vi "Read_ROI.vi"(8 "error in":errorcluster, 11 "Experiment folder path":path) -> (0 "error out":errorcluster, 2 "ROI setup":T1[](array[typedef]) {"ROI group ID" format="%#_6f"; "Laser Power (%)" format="%#_6f"; "Zoom" format="%#_6f"; "Frame Size" format="%#_6f"; "Number of lines" format="%#_6f"; "Composite ID" format="%#_6f"; "Angle (deg)" format="%#_6f"; "ROI Time (ns)" format="%#_6f"; "ROI ID" format="%#_6f"; "Pixels in ROI" format="%#_6f"; "ROI index" format="%#_6f"; "Z stop" format="%#_6f"; "Y stop" format="%#_6f"; "X stop" format="%#_6f"; "Z start" format="%#_6f"; "X start" format="%#_6f"; "Y start" format="%#_6f"})   [LabVIEW 2013]
uses:
  User Interface/Visualisation/Functional Imaging Viewer/Typedefs/ROI parameters data type.ctl
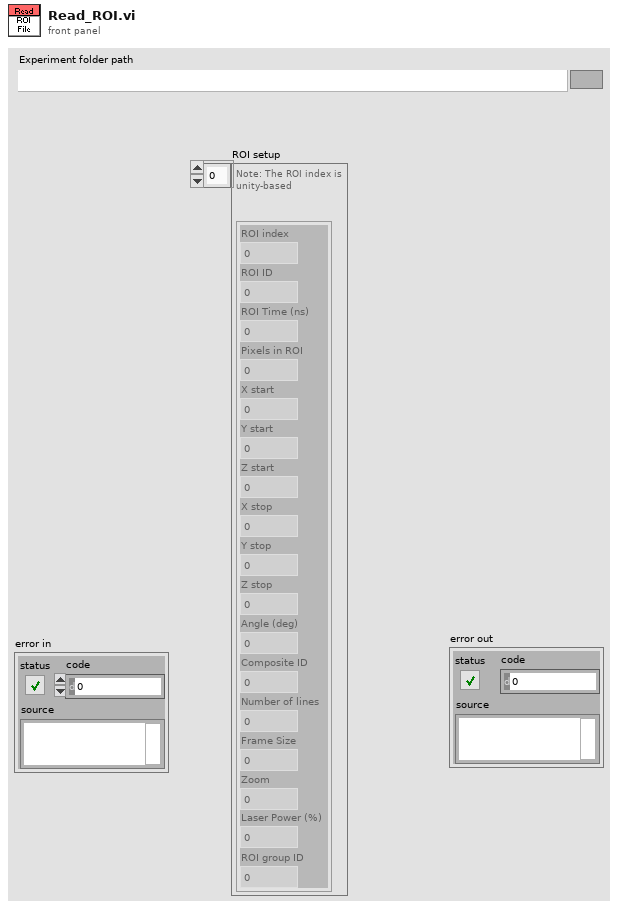
[diagram p1: front panel]
types:
  T1 = typedef "ROI parameters data type.ctl" = cluster{"ROI index":dbl, "ROI ID":dbl, "ROI Time (ns)":dbl, "Pixels in ROI":dbl, "X start":dbl, "Y start":dbl, "Z start":dbl, "X stop":dbl, "Y stop":dbl, "Z stop":dbl, "Angle (deg)":dbl, "Composite ID":dbl, "Number of lines":dbl, "Frame Size":dbl, "Zoom":dbl, "Laser Power (%)":dbl, "ROI group ID":dbl}
  T2 = typedef "Fixed strings.ctl" = cluster{"ROI file name":string, "Normalised ROI file name":string, "Zplane Pockels values file name":string, "Functional data folder name":string, "Experiment Header file name":string, "Z-stack images folder name":string, "Groups setup rel. path":string, "Groups text file rel. path":string, "TDMS files folder name (F.img)":string, "TDMS files folder name (V.acq)":string, "TDMS files folder name (Pl.acq)":string, "Cycle rel times sequence file":string, "Dynamically called VIs folder name":string, "Time Series folder base name":string}
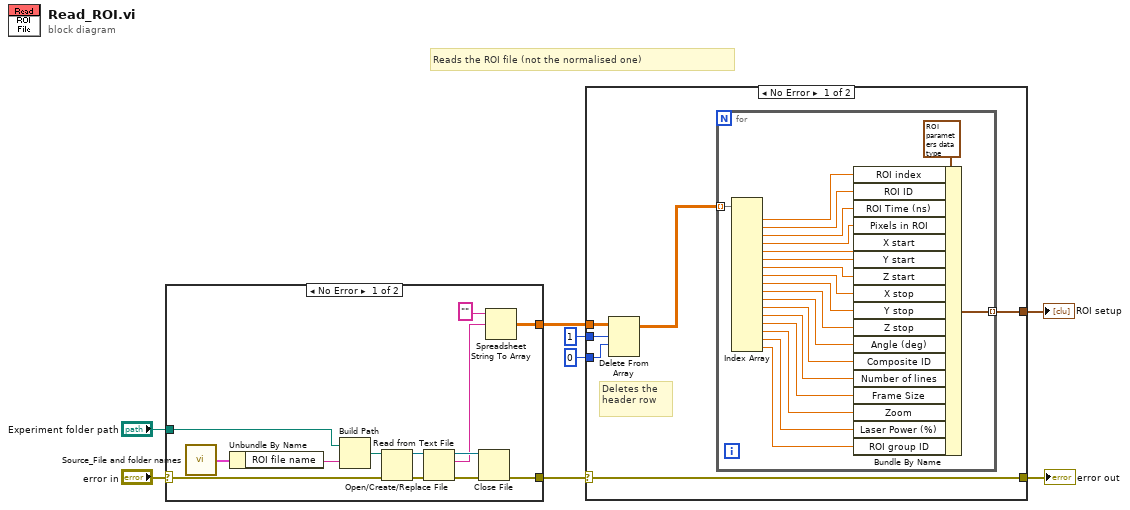
[diagram p0: block diagram]
diagram:
  # "Reads the ROI file (not the normalised one)"
  n1 = case shown="No Error" "error in" {
    selector: "error in" -> [w13 w22]
    tunnel: [w14 _] -> w8
    tunnel: [w12 w22] -> w4
    tunnel: "Experiment folder path" -> [w11 _]
    frame No Error {
      n2 = call "Source_File and folder names.vi"() -> ("Fixed strings"=w10:T2)  [unwired: 1 in]
      n3 = Unbundle By Name(w10) -> ("ROI file name"=w9:string)
      n4 = Build Path(base path=w11, name or relative path=w9) -> (appended path=w21:path)
      n5 = Open/Create/Replace File(file path (use dialog)=w21, error in=w13) -> (refnum out=w20:refnum<file>, error out=w19:errorcluster)  [unwired: 4 in, 1 out]
      n6 = Read from Text File(file (use dialog)=w20, error in=w19) -> (refnum out=w18:refnum<file>, text=w16:string, error out=w17:errorcluster)  [unwired: 2 in, 1 out]
      n7 = Close File(refnum=w18, error in=w17) -> (error out=w12:errorcluster)  [unwired: 1 out]
      n8 = Spreadsheet String To Array(format string="", spreadsheet string=w16) -> (array=w14:dbl[][])  [unwired: 2 in]
    }
    frame Error {
    }
  }
  n9 = case shown="No Error" w4 {
    selector: w4 -> [w25 w49]
    tunnel: w8 -> [w24 _]
    tunnel: 1 ("length") -> [w28 _]
    tunnel: 0 ("index (row)") -> [w27 _]
    tunnel: [w25 w49] -> w3
    tunnel: [w23 _] -> w1
    frame No Error {
      # "Deletes the header row"
      n10 = Delete From Array "Delete From Array"(array=w24, length=w28, index (row)=w27) -> (array with subset deleted=w26:dbl[][])  [unwired: 1 in, 1 out]
      n11 = for {
        tunnel: w26 -> [w48] mode=indexing
        tunnel: [w38] -> w23 mode=indexing
        n12 = Index Array(array=w48) -> (element #1=w47:dbl, element #2=w46:dbl, element #3=w45:dbl, element #4=w44:dbl, element #5=w43:dbl, element #6=w42:dbl, element #7=w41:dbl, element #8=w40:dbl, element #9=w39:dbl, element #10=w36:dbl, element #11=w35:dbl, element #12=w34:dbl, element #13=w33:dbl, element #14=w32:dbl, element #15=w31:dbl, element #16=w30:dbl, element #17=w29:dbl)  [unwired: 17 in]
        n13 = Bundle By Name(cluster=T1 {"ROI index"=0.0, "ROI ID"=0.0, "ROI Time (ns)"=0.0, "Pixels in ROI"=0.0, "X start"=0.0, "Y start"=0.0, "Z start"=0.0, "X stop"=0.0, "Y stop"=0.0, "Z stop"=0.0, "Angle (deg)"=0.0, "Composite ID"=0.0, "Number of lines"=0.0, "Frame Size"=0.0, "Zoom"=0.0, "Laser Power (%)"=0.0, "ROI group ID"=0.0} ("X-Y-Z coordinates"), "ROI index"=w47, "ROI ID"=w46, "ROI Time (ns)"=w45, "Pixels in ROI"=w44, "X start"=w43, "Y start"=w42, "Z start"=w41, "X stop"=w40, "Y stop"=w39, "Z stop"=w36, "Angle (deg)"=w35, "Composite ID"=w34, "Number of lines"=w33, "Frame Size"=w32, "Zoom"=w31, "Laser Power (%)"=w30, "ROI group ID"=w29) -> (w38:T1)
      }
    }
    frame Error {
    }
  }
  "error out" <- w3
  "ROI setup" <- w1
